vi "Read Weight.vi"(8 "error in (no error)":errorcluster, 11 "Instrument.LN2 in":refnum<class "Instrument.LN2.lvclass">) -> (0 "error out":errorcluster, 2 "Weight":dbl, 3 "Instrument.LN2 out":refnum<class "Instrument.LN2.lvclass">)   [LabVIEW 2019, in "Instrument.LN2.lvclass"]
uses:
  Instrument.LN2.lvclass
  Instrument.LN2.lvclass/Instrument.LN2.ctl
  <vilib>/regexp/Match Regular Expression.xnode
panel:
  in  "stop":bool
  out "before match":string
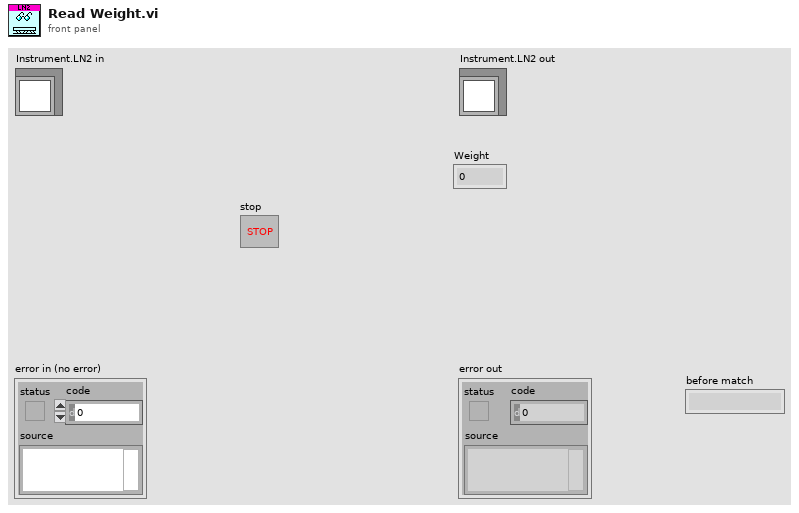
[diagram p1: front panel]
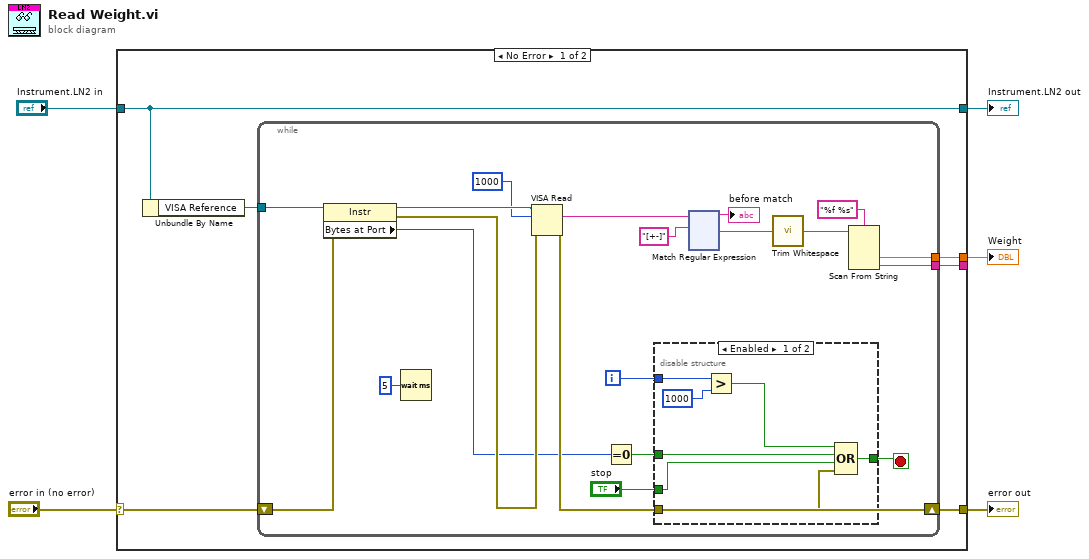
[diagram p0: block diagram]
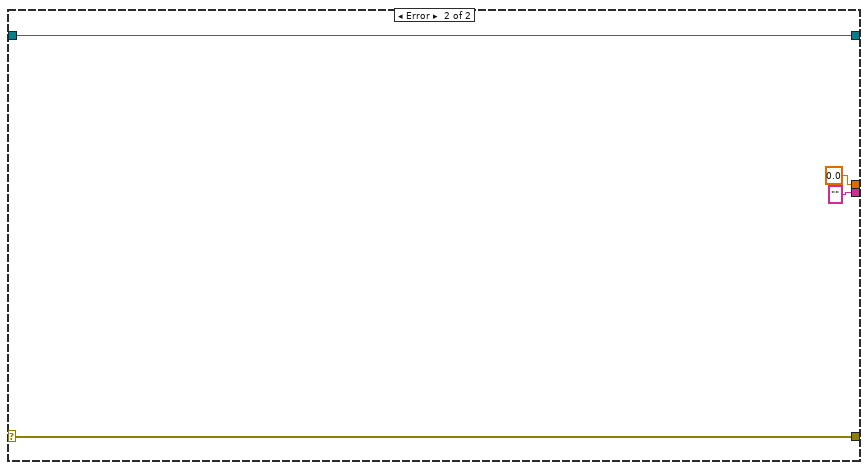
[diagram p3: hidden frame]
diagram:
  n1 = case shown="No Error" "error in (no error)" {
    selector: "error in (no error)" -> [w8 w157]
    tunnel: [w11 w157] -> w4
    tunnel: [w7 w156] -> w2
    tunnel: "Instrument.LN2 in" -> [w7 w156]
    tunnel: [w10 0.0] -> w1
    tunnel: [w6 ""] -> _
    frame No Error {
      n2 = Unbundle By Name(w7) -> ("VISA Reference"=w9:refnum<visa-resource-name>)
      n3 = while {
        tunnel: w9 -> [w31]
        tunnel: [w23] -> w10
        shift-right: [w16] -> w11
        shift-left: w8 -> [w21]
        tunnel: [w14] -> w6
        i -> [w15]
        stop <- w18 stop-if-true
        n4 = property class="Instr"(reference=w31, error in=w21) -> (reference out=w30:refnum<visa-resource-name>, error out=w22:errorcluster, "Bytes at Port"=w12:u32)
        n5 = Wait (ms)(milliseconds to wait=u32 5) -> ()  [unwired: 1 out]
        n6 = VISA Read(VISA resource name=w30, byte count=u32 1000, error in (no error)=w22) -> (read buffer=w26:string, error out=w16:errorcluster)  [unwired: 2 out]
        n7 = Equal To 0?(x=w12) -> (x = 0?=w19:bool)
        n8 = disable-structure shown="Enabled" {
          disable-tunnel: w19 -> [w38 _]
          disable-tunnel: [w37 w39] -> w18
          disable-tunnel: w16 -> [w36 _]
          disable-tunnel: w15 -> [w35 _]
          disable-tunnel: "stop" -> [w32 w39]
          frame Enabled {
            n9 = Greater?(x=w35, y=1000) -> (0:w33:bool)
            n10 = Compound Arithmetic op=OR(w33, w38, w32, w36) -> (w37:bool)
          }
          frame Disabled {
          }
        }
        n11 = xnode "Match Regular Expression"("input string"=w26, "regular expression"="[+-]" ("format string")) -> ("before match"=→"before match":string, "after match"=w25:string)  [unwired: 4 in, 3 out]
        n12 = call <vilib>:"Trim Whitespace.vi"("string"=w25) -> ("trimmed string"=w24:string)  [unwired: 1 in]
        n13 = Scan From String(format string="%f %s", input string=w24) -> (output 1=w23:dbl, output 2=w14:string)  [unwired: 4 in, 3 out]
      }
    }
    frame Error {
    }
  }
  "error out" <- w4
  "Instrument.LN2 out" <- w2
  "Weight" <- w1
